vi "Init Caraya Test Suite.vi"(8 "error in (no error)":errorcluster, 10 "Properties.Suite":refnum<class "Properties.Suite.lvclass">, 11 "TestSuite":refnum<class "Test Suite.lvclass">) -> (0 "error out":errorcluster, 2 "Leaf.Properties.TestSuite out":refnum<class "Leaf.Properties.Suite.lvclass">, 3 "Platano.CarayaTestSuite out":refnum<class "Platano.CarayaTestSuite.lvclass">)   [LabVIEW 2021, in "Banana.Caraya.lvlib" / "Platano.CarayaTestSuite.lvclass"]
uses:
  Platano.CarayaTestSuite.lvclass
  <vilib>/addons/_JKI Toolkits/Caraya/classes/Test Suite/Test Suite.lvclass
  <vilib>/addons/_JKI Toolkits/Caraya/classes/Properties.Suite/Properties.Suite.lvclass
  Leaf.Properties.Suite/Leaf.Properties.Suite.lvclass
  C:/Repositories/LVOS/Bananas/lv-src/Bananas/Leaf/Leaf.lvclass
  Platano.CarayaTestSuite.lvclass/Platano.CarayaTestSuite.ctl
  Bananas/Leaf/Leaf.lvclass
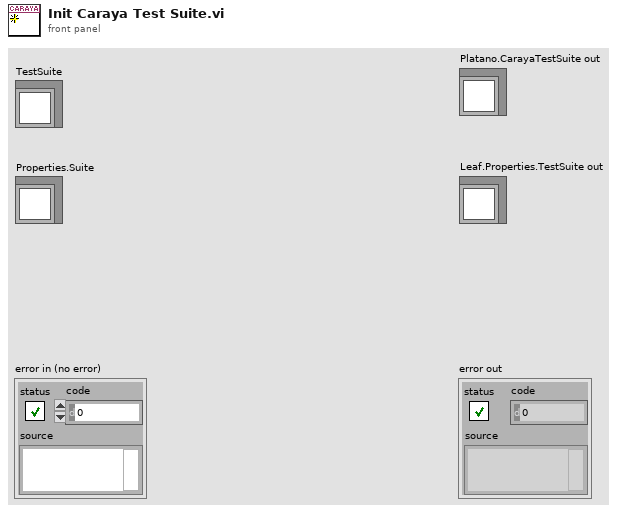
[diagram p1: front panel]
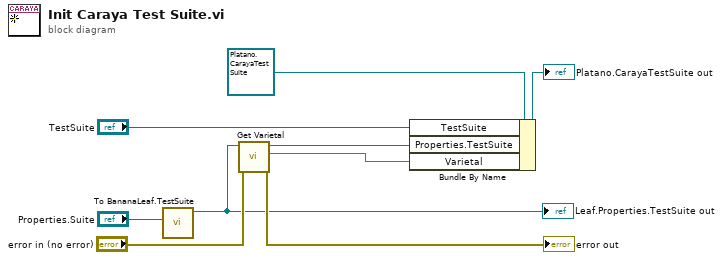
[diagram p0: block diagram]
diagram:
  n1 = call "To BananaLeaf.TestSuite.vi"("Properties.Suite"="Properties.Suite") -> ("Leaf.Properties.TestSuite out"=w1:refnum<class "Leaf.Properties.Suite.lvclass">)  [unwired: 10 in]
  "Leaf.Properties.TestSuite out" <- w1
  n2 = call "Get Varietal.vi"("error in (no error)"="error in (no error)", "Leaf in"=w1) -> ("error out"=→"error out":errorcluster, "Varietal"=w6:string, "Leaf out"=w5:refnum<class "Leaf.Properties.Suite.lvclass">)  [unwired: 7 in]
  n3 = Bundle By Name(cluster=refnum<class "Platano.CarayaTestSuite.lvclass"> refnum ("Platano.CarayaTestSuite in"), "TestSuite"="TestSuite", "Properties.TestSuite"=w5, "Varietal"=w6) -> (→"Platano.CarayaTestSuite out":refnum<class "Platano.CarayaTestSuite.lvclass">)
